vi "finish_waypoint.vi"(11 "Waypoint in":refnum<class "Waypoint.lvclass">) -> (3 "Waypoint out":refnum<class "Waypoint.lvclass">)   [LabVIEW 2011, in "Waypoint.lvclass"]
uses:
  Waypoint.lvclass
  Waypoint.lvclass/Waypoint.ctl
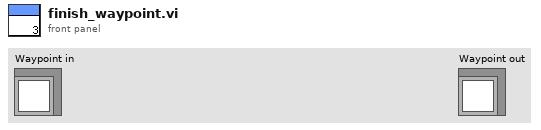
[diagram p1: front panel]
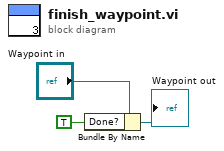
[diagram p0: block diagram]
diagram:
  n1 = Bundle By Name(cluster="Waypoint in", "Done?"=TRUE) -> (→"Waypoint out":refnum<class "Waypoint.lvclass">)
